vi "ProgressCmdResponse512.vi"(0 "connection ID control":refnum<k5>, 1 "Command for FW upgrade":string="1||1||1||AC.bin||PC.bin||SC.bin", 5 "FW Message ID":i32, 7 "FW Message Length":i32, 8 "Response ID 1":u8, 9 "error in (no error)":errorcluster, 17 "Time Delay":i16=10) -> (20 "connection ID":refnum<k5>, 22 "AC-FW upgrade pregress bar":u8(slide) scale=0.0..100.0, 23 "PC-FW upgrade pregress bar":u8(slide) scale=0.0..100.0, 24 "SC-FW upgrade pregress bar":u8(slide) scale=0.0..100.0, 25 "error out":errorcluster, 27 "Pass":string="Horn Scan Success")   [LabVIEW 2017]
panel:
  out "Firware Upgrade response":string
  out "*(type *) &x":u8
  out "rest of the binary string":string
  out "Message Length":u8
  out "Message ID":u8
  out "bytes written":i32
  # "Input"
  # "For Info:\nAC=1 Upgrade required, 0 Upgrade not required\nPC=1 Upgrade required, 0 Upgrade not required\nSC=1 Upgrade required, 0 Upgrade not required"
  # "Output"
  # "Refrence:"
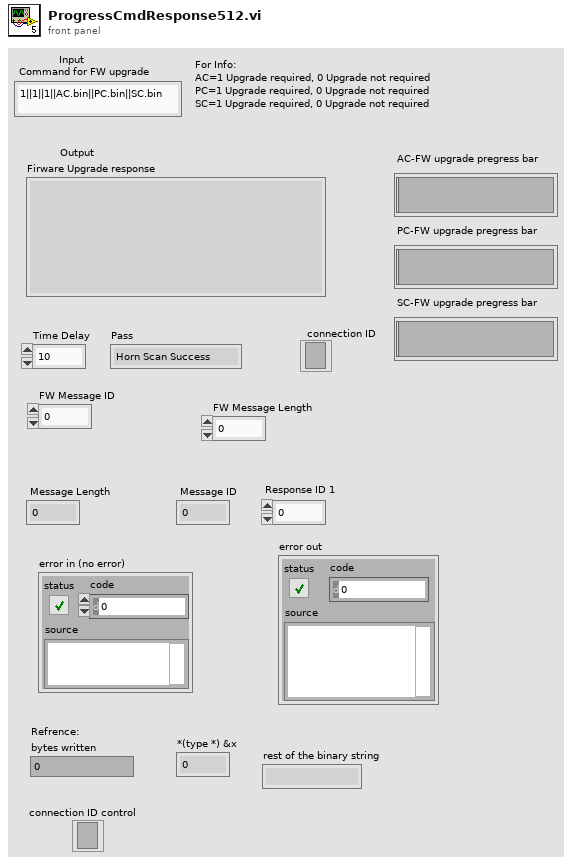
[diagram p1: front panel]
types:
  T1 = enum16{"big-endian, network order", "native, host order", "little-endian"}
  T2 = cluster{"Command for FW upgrade":string, "FW Message Length":i32, "FW Message ID":i32}
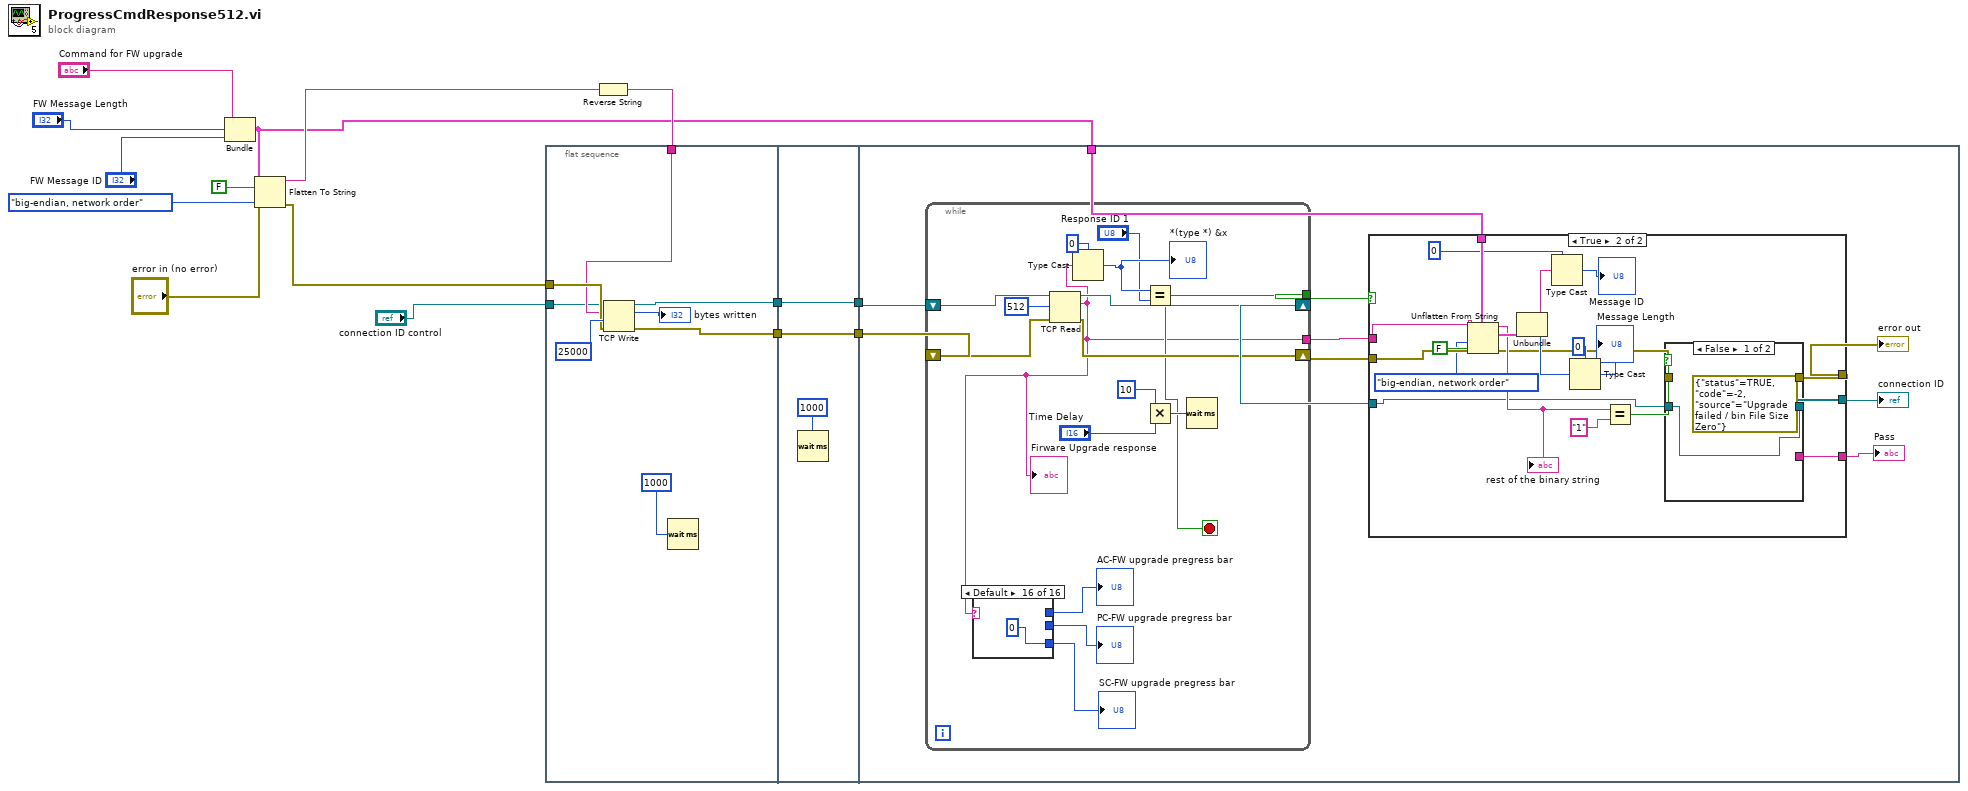
[diagram p0: block diagram]
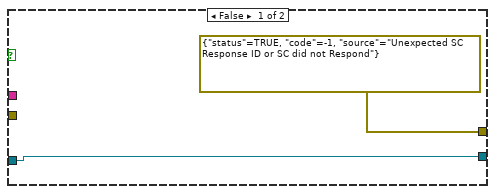
[diagram p2: hidden frame]
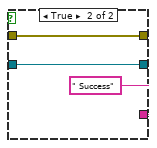
[diagram p3: hidden frame]
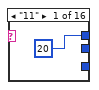
[diagram p4: hidden frame]
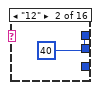
[diagram p5: hidden frame]
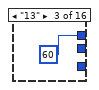
[diagram p6: hidden frame]
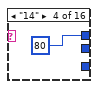
[diagram p7: hidden frame]
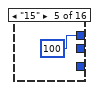
[diagram p8: hidden frame]
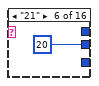
[diagram p9: hidden frame]
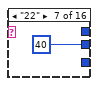
[diagram p10: hidden frame]
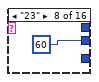
[diagram p11: hidden frame]
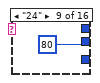
[diagram p12: hidden frame]
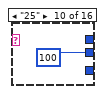
[diagram p13: hidden frame]
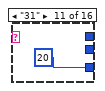
[diagram p14: hidden frame]
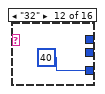
[diagram p15: hidden frame]
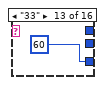
[diagram p16: hidden frame]
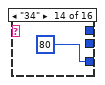
[diagram p17: hidden frame]
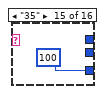
[diagram p18: hidden frame]
diagram:
  n1 = Bundle("Command for FW upgrade"="Command for FW upgrade", "FW Message Length"="FW Message Length", "FW Message ID"="FW Message ID") -> (w4:T2)  [unwired: 1 in]
  n2 = Flatten To String(anything=w4, prepend array or string size? (T)=FALSE, byte order (0:big-endian, network order)=T1."big-endian, network order", error in (no error)="error in (no error)") -> (data string=w7:string, error out=w8:errorcluster)  [unwired: 1 out]
  n3 = flat-sequence {
    tunnel: [w21] -> w15
    tunnel: [w20] -> w14
    tunnel: w8 -> [w19]
    tunnel: w6 -> [w18]
    tunnel: "connection ID control" -> [w16]
    tunnel: [w25] -> w13
    tunnel: w15 -> [w25]
    tunnel: [w24] -> w12
    tunnel: w14 -> [w24]
    tunnel: w13 -> [w36]
    tunnel: w12 -> [w35]
    tunnel: w4 -> [w34]
    frame #0 {
      n4 = TCP Write(connection ID=w16, data in=w18, error in (no error)=w19, 9:25000 ("timeout ms (25000)")) -> (connection ID out=w21:refnum<k5>, bytes written=→"bytes written":i32, error out=w20:errorcluster)
      n5 = Wait (ms)(milliseconds to wait=u32 1000) -> ()  [unwired: 1 out]
    }
    frame #1 {
      n6 = Wait (ms)(milliseconds to wait=u32 1000) -> ()  [unwired: 1 out]
    }
    frame #2 {
      n7 = while {
        tunnel: [w64] -> w33
        shift-right: [w77] -> w29
        shift-left: w36 -> [w79]
        shift-right: [w75] -> w32
        shift-left: w35 -> [w78]
        tunnel: [w68] -> w31
        stop <- w68 stop-if-true
        n8 = TCP Read(connection ID=w79, bytes to read=512, error in (no error)=w78) -> (connection ID out=w77:refnum<k5>, data out=w64:string, error out=w75:errorcluster)  [unwired: 2 in]
        "Firware Upgrade response" <- w64
        n9 = case shown="Default" w64 {
          tunnel: [20 40 60 80 100 _ _ _ _ _ _ _ _ _ _ _] -> w67
          tunnel: [_ _ _ _ _ 20 40 60 80 100 _ _ _ _ _ _] -> w66
          tunnel: [_ _ _ _ _ _ _ _ _ _ 20 40 60 80 100 0] -> w65
          frame "11" {
          }
          frame "12" {
          }
          frame "13" {
          }
          frame "14" {
          }
          frame "15" {
          }
          frame "21" {
          }
          frame "22" {
          }
          frame "23" {
          }
          frame "24" {
          }
          frame "25" {
          }
          frame "31" {
          }
          frame "32" {
          }
          frame "33" {
          }
          frame "34" {
          }
          frame "35" {
          }
          frame Default {
          }
        }
        "AC-FW upgrade pregress bar" <- w67
        "PC-FW upgrade pregress bar" <- w66
        "SC-FW upgrade pregress bar" <- w65
        n10 = Type Cast(type=u8 0, x=w64) -> (*(type *) &x=w73:u8)
        "*(type *) &x" <- w73
        n11 = Equal?(x=w73, y="Response ID 1") -> (x = y?=w68:bool)
        n12 = Multiply(x=i16 10 ("milliseconds to wait"), y="Time Delay") -> (x*y=w70:i16)
        n13 = Wait (ms)(milliseconds to wait=w70) -> ()  [unwired: 1 out]
      }
      n14 = case shown="True" w31 {
        tunnel: w34 -> [_ w57]
        tunnel: w33 -> [_ w49]
        tunnel: w32 -> [_ w48]
        tunnel: [w38 w40] -> w30
        tunnel: w29 -> [w38 w41]
        tunnel: [errorcluster {"status"=TRUE, "code"=-1, "source"="Unexpected SC Response ID or SC did not Respond"} ("error constant") w42] -> w28
        tunnel: [_ w39] -> w27
        frame False {
        }
        frame True {
          n15 = Unflatten From String(type=w57, binary string=w49, data includes array or string size? (T)=FALSE, byte order (0:big-endian, network order)=T1."big-endian, network order", error in (no error)=w48) -> (rest of the binary string=w46:string, value=w58:T2, error out=w43:errorcluster)
          "rest of the binary string" <- w46
          n16 = Unbundle(w58) -> ("Command for FW upgrade"=w51:string, "FW Message Length"=w55:i32)  [unwired: 1 out]
          n17 = Type Cast(type=u8 0, x=w51) -> (*(type *) &x=→"Message ID":u8)
          n18 = Type Cast(type=u8 0, x=w55) -> (*(type *) &x=→"Message Length":u8)
          n19 = Equal?(x=w46, y="1") -> (x = y?=w44:bool)
          n20 = case shown="False" w44 {
            tunnel: w43 -> [_ w63]
            tunnel: [errorcluster {"status"=TRUE, "code"=-2, "source"="Upgrade failed / bin File Size Zero"} ("error constant") w63] -> w42
            tunnel: w41 -> [w59 w62]
            tunnel: [w59 w62] -> w40
            tunnel: [_ " Success"] -> w39
            frame False {
            }
            frame True {
            }
          }
        }
      }
      "error out" <- w28
      "connection ID" <- w30
      "Pass" <- w27
    }
  }
  n21 = Reverse String(1:w7) -> (0:w6:string)
